vi "gCode_AnalizeAndSend.vi"(9 "UI_Data":T1={"controlTabState"=[], "pathToSTLFiles"=path "", "availableObjs"=[], "objectNames"=[], "addedObjs"=[], "selectedObj"={"Name"="", "objectFiles"=[], "center"={"X"=0.0, "Y"=0.0, "Z"=0.0}, "extent"={"X"=0.0, "Y"=0.0, "Z"=0.0}, "allowedMotion"=enum."XY", "mountOn"=enum."yArm", "Movements"=[], "extraInfo"=[], "hasPOI?"=FALSE, "POI"={"X"=0.0, "Y"=0.0, "Z"=0.0}, "posOffset"={"X"=0.0, "Y"=0.0, "Z"=0.0}, "referenceNum"=refnum}, "3DPictureObjRef"=refnum, "yPOI_0"={"X"=0.0, "Y"=0.0, "Z"=0.0}, "yPOI"={"X"=0.0, "Y"=0.0, "Z"=0.0}, "yPOI_Added?"=FALSE, "breadBoard_00"={"X"=0.0, "Y"=0.0, "Z"=0.0}, "breadBoardOriginOffset"={"X"=0.0, "Y"=0.0, "Z"=0.0}, "XYtranslateObjControls"=[], "ZtranslateObjControls"=[], "pBot_controls"=[], "pBot_VISA"="", "commandLog"="", "pBotConnected?"=FALSE, "pBot_currentEEPROMsettings"="", "realTimeInfoControls"=[], "pBot_tempSensor1"=0.0, "pBot_tempSensor2"=0.0, "realTimeInfoTextColor"=[], "disconnectPBot_Event"=refnum, "needToHomeY?"=FALSE, "pBot_relativePositioning"=FALSE, "pBot_minPos"={"X"=0.0, "Y"=0.0, "Z"=0.0}, "pBot_maxPos"={"X"=0.0, "Y"=0.0, "Z"=0.0}, "pBot_homeOffset"={"X"=0.0, "Y"=0.0, "Z"=0.0}, "textColorGreen"=9174826, "textColorRed"=16750216, "textColorGray"=9868950, "transVisualizationControls"=[], "needToHomeXY?"=FALSE, "pBot_minScanRegion"={"X"=0.0, "Y"=0.0, "Z"=0.0}, "pBot_maxScanRegion"={"X"=0.0, "Y"=0.0, "Z"=0.0}, "pBot_scanN"={"X"=0, "Y"=0, "Z"=0}, "connectedInstruments"=[], "isScanning?"=FALSE, "Wavelengths"=[], "usb2000p_controlRefs"=[], "3DPictureRef"=refnum}, 10 "Input String":string, 11 "Equip_Queue":refnum<queue>) -> (0 "errorOut":errorcluster, 1 "UI_Data out":T1={"controlTabState"=[], "pathToSTLFiles"=path "", "availableObjs"=[], "objectNames"=[], "addedObjs"=[], "selectedObj"={"Name"="", "objectFiles"=[], "center"={"X"=0.0, "Y"=0.0, "Z"=0.0}, "extent"={"X"=0.0, "Y"=0.0, "Z"=0.0}, "allowedMotion"=enum."XY", "mountOn"=enum."yArm", "Movements"=[], "extraInfo"=[], "hasPOI?"=FALSE, "POI"={"X"=0.0, "Y"=0.0, "Z"=0.0}, "posOffset"={"X"=0.0, "Y"=0.0, "Z"=0.0}, "referenceNum"=refnum}, "3DPictureObjRef"=refnum, "yPOI_0"={"X"=0.0, "Y"=0.0, "Z"=0.0}, "yPOI"={"X"=0.0, "Y"=0.0, "Z"=0.0}, "yPOI_Added?"=FALSE, "breadBoard_00"={"X"=0.0, "Y"=0.0, "Z"=0.0}, "breadBoardOriginOffset"={"X"=25.4, "Y"=12.7, "Z"=12.7}, "XYtranslateObjControls"=[], "ZtranslateObjControls"=[], "pBot_controls"=[], "pBot_VISA"="", "commandLog"="", "pBotConnected?"=FALSE, "pBot_currentEEPROMsettings"="", "realTimeInfoControls"=[], "pBot_tempSensor1"=0.0, "pBot_tempSensor2"=0.0, "realTimeInfoTextColor"=[], "disconnectPBot_Event"=refnum, "needToHomeY?"=FALSE, "pBot_relativePositioning"=FALSE, "pBot_minPos"={"X"=0.0, "Y"=0.0, "Z"=0.0}, "pBot_maxPos"={"X"=0.0, "Y"=0.0, "Z"=0.0}, "pBot_homeOffset"={"X"=0.0, "Y"=0.0, "Z"=0.0}, "textColorGreen"=9174826, "textColorRed"=16750216, "textColorGray"=9868950, "transVisualizationControls"=[], "needToHomeXY?"=FALSE, "pBot_minScanRegion"={"X"=0.0, "Y"=0.0, "Z"=0.0}, "pBot_maxScanRegion"={"X"=0.0, "Y"=0.0, "Z"=0.0}, "pBot_scanN"={"X"=0, "Y"=0, "Z"=0}, "connectedInstruments"=[], "isScanning?"=FALSE, "Wavelengths"=[], "usb2000p_controlRefs"=[], "3DPictureRef"=refnum})   [LabVIEW 2015]
uses:
  controls/UI Data.ctl
  processedObjectInfo.ctl
  controls/scanInstrumentInfo.ctl
  support/Message Queue/Message Cluster.ctl
  controls/pBotMessageData.ctl
  support/Message Queue/Enqueue Message (Single).vi
  support/Message Queue/Message Queue.lvlib
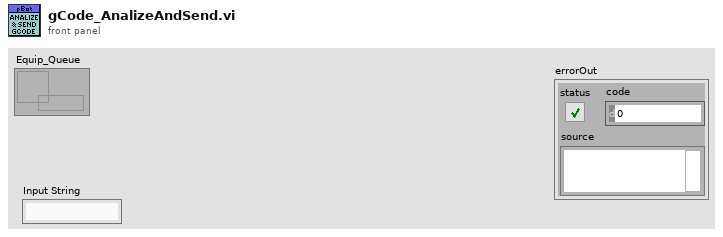
[diagram p1: front panel]
types:
  T1 = typedef "UI Data.ctl" = cluster{"controlTabState":bool[], "pathToSTLFiles":path, "availableObjs":T2[], "objectNames":string[], "addedObjs":T2[], "selectedObj":T2, "3DPictureObjRef":refnum<vi>, "yPOI_0":cluster{"X":dbl, "Y":dbl, "Z":dbl}, "yPOI":cluster{"X":dbl, "Y":dbl, "Z":dbl}, "yPOI_Added?":bool, "breadBoard_00":cluster{"X":dbl, "Y":dbl, "Z":dbl}, "breadBoardOriginOffset":cluster{"X":dbl, "Y":dbl, "Z":dbl}, "XYtranslateObjControls":refnum<vi>[], "ZtranslateObjControls":refnum<vi>[], "pBot_controls":refnum<vi>[], "pBot_VISA":refnum<visa-resource-name>, "commandLog":string, "pBotConnected?":bool, "pBot_currentEEPROMsettings":string, "realTimeInfoControls":refnum<vi>[], "pBot_tempSensor1":dbl, "pBot_tempSensor2":dbl, "realTimeInfoTextColor":u32[], "disconnectPBot_Event":refnum<user-event>, "needToHomeY?":bool, "pBot_relativePositioning":bool, "pBot_minPos":cluster{"X":dbl, "Y":dbl, "Z":dbl}, "pBot_maxPos":cluster{"X":dbl, "Y":dbl, "Z":dbl}, "pBot_homeOffset":cluster{"X":dbl, "Y":dbl, "Z":dbl}, "textColorGreen":u32, "textColorRed":u32, "textColorGray":u32, "transVisualizationControls":refnum<vi>[], "needToHomeXY?":bool, "pBot_minScanRegion":cluster{"X":sgl, "Y":sgl, "Z":sgl}, "pBot_maxScanRegion":cluster{"X":sgl, "Y":sgl, "Z":sgl}, "pBot_scanN":cluster{"X":u16, "Y":u16, "Z":u16}, "connectedInstruments":T3[], "isScanning?":bool, "Wavelengths":dbl[], "usb2000p_controlRefs":refnum<vi>[], "3DPictureRef":refnum<vi>}
  T2 = typedef "processedObjectInfo.ctl" = cluster{"Name":string, "objectFiles":cluster{"Location":path, "Color":cluster{"R":dbl, "G":dbl, "B":dbl, "A":dbl}}[], "center":cluster{"X":dbl, "Y":dbl, "Z":dbl}, "extent":cluster{"X":dbl, "Y":dbl, "Z":dbl}, "allowedMotion":enum16{"XY", "Z"}, "mountOn":enum16{"yArm", "breadBoard"}, "Movements":cluster{"Type":enum16{"rr", "ra", "tr", "ta"}, "vector":cluster{"X":dbl, "Y":dbl, "Z":dbl}, "scalar":dbl}[], "extraInfo":cluster{"parameter":string, "dataType":string, "vector":cluster{"X":dbl, "Y":dbl, "Z":dbl}, "scalar":dbl}[], "hasPOI?":bool, "POI":cluster{"X":dbl, "Y":dbl, "Z":dbl}, "posOffset":cluster{"X":dbl, "Y":dbl, "Z":dbl}, "referenceNum":refnum<vi>}
  T3 = typedef "scanInstrumentInfo.ctl" = cluster{"Name":string, "VISAname":refnum<visa-resource-name>, "1D_dataArraySize":u16, "extraInfo":variant, "error":errorcluster}
  T4 = typedef "pBotMessageData.ctl" = cluster{"commandID":string, "gCode":string, "extraInfo":string, "originatingCommandID":string, "error":errorcluster}
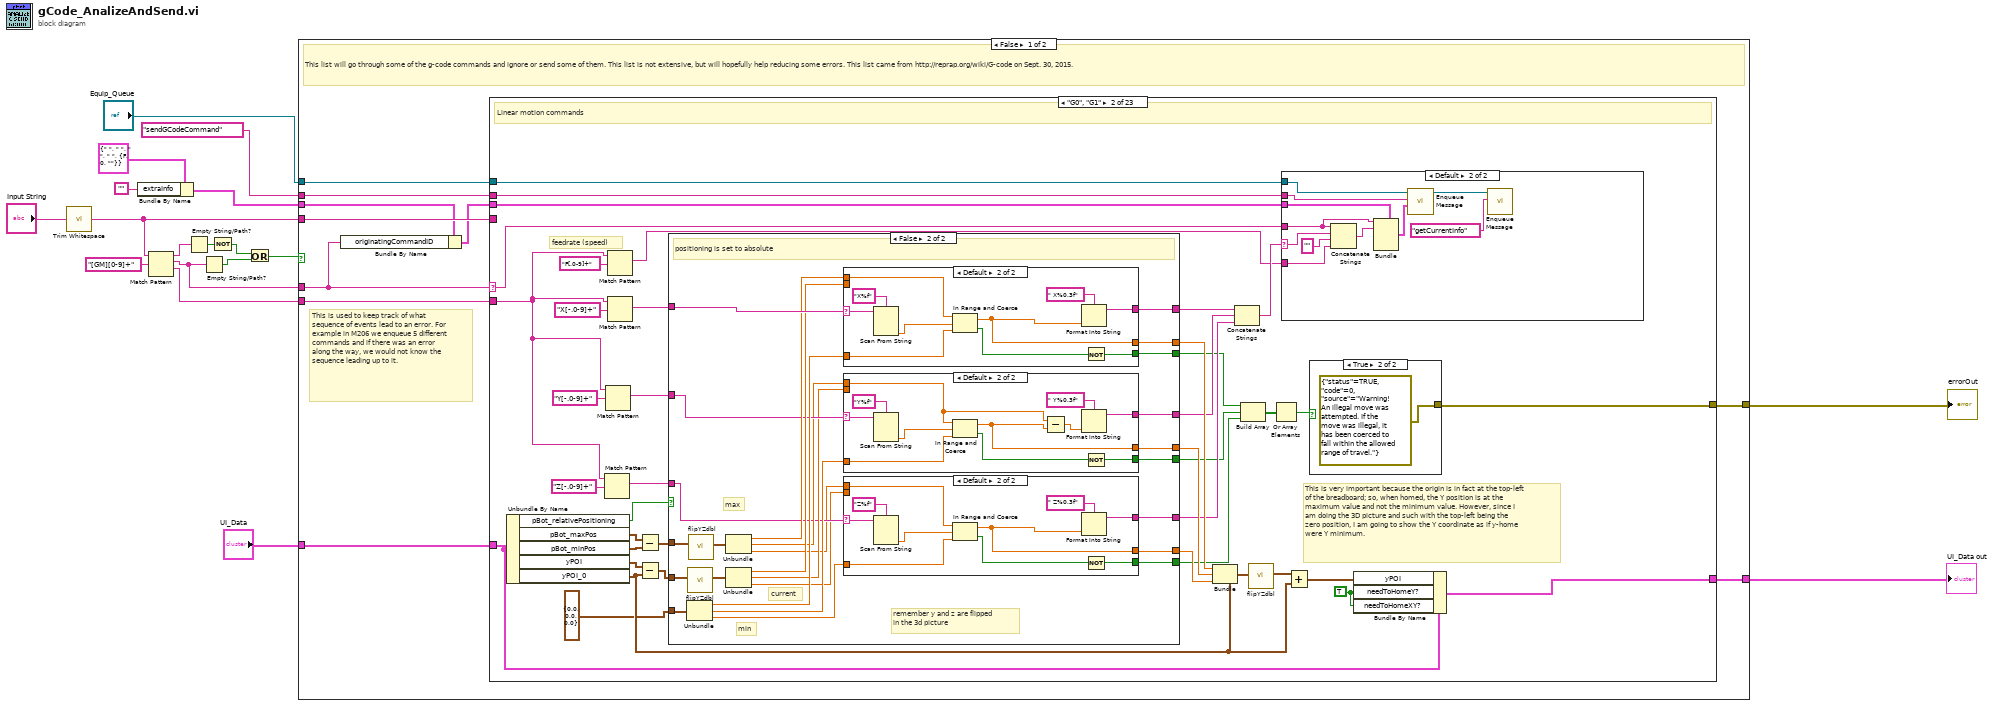
[diagram p0: block diagram]
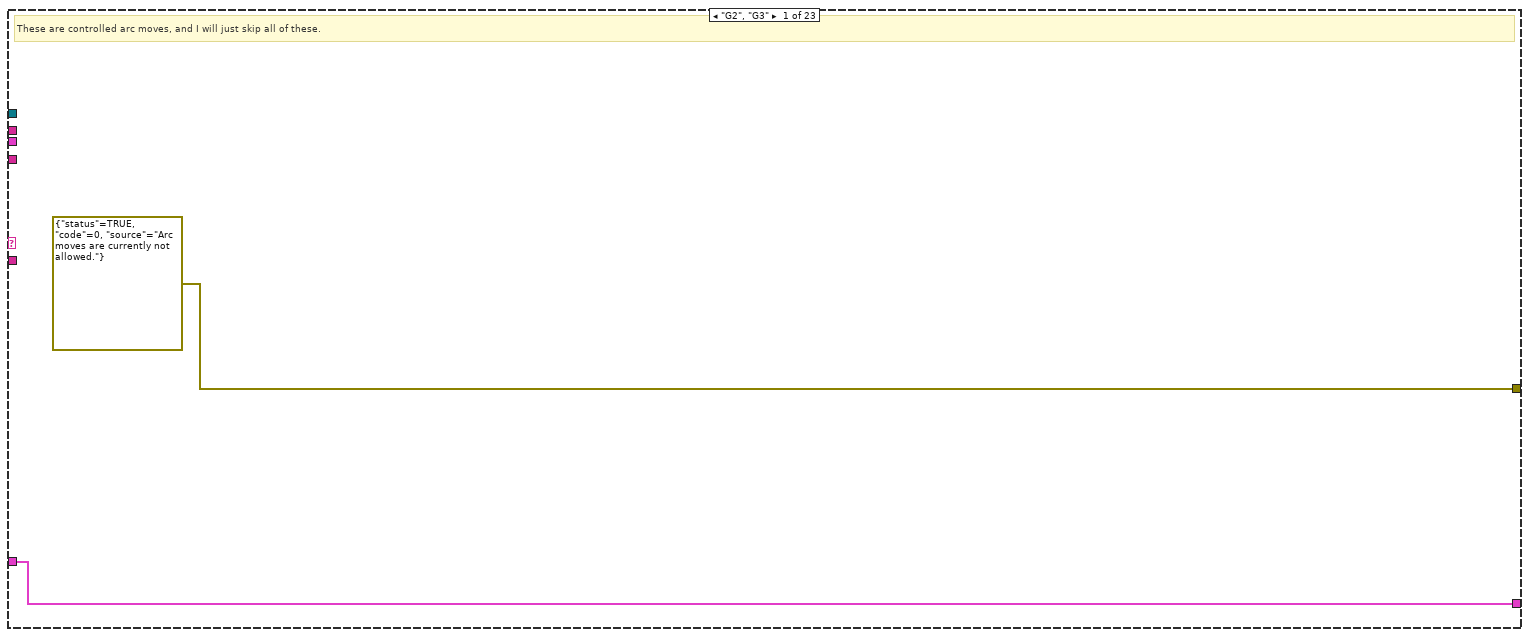
[diagram p2: hidden frame]
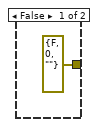
[diagram p3: hidden frame]
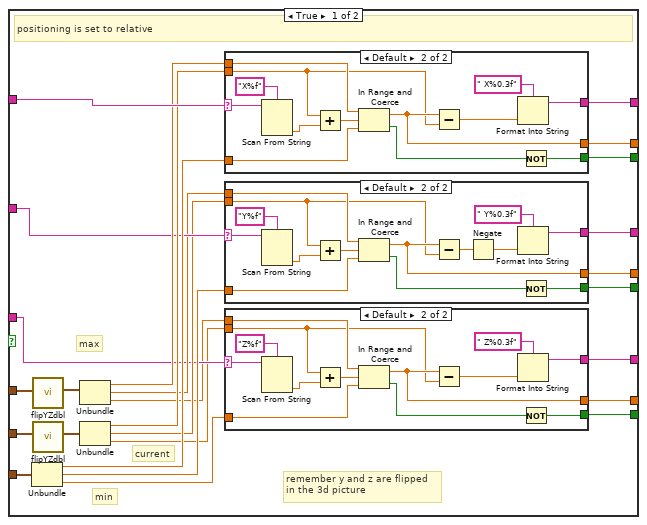
[diagram p5: hidden frame]
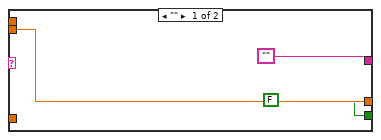
[diagram p6: hidden frame]
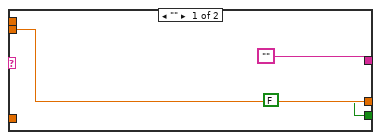
[diagram p7: hidden frame]
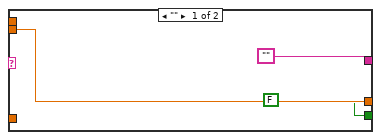
[diagram p8: hidden frame]
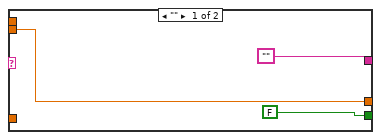
[diagram p9: hidden frame]
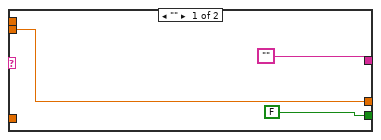
[diagram p10: hidden frame]
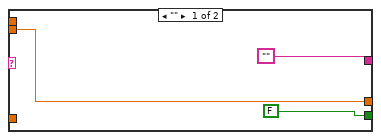
[diagram p11: hidden frame]
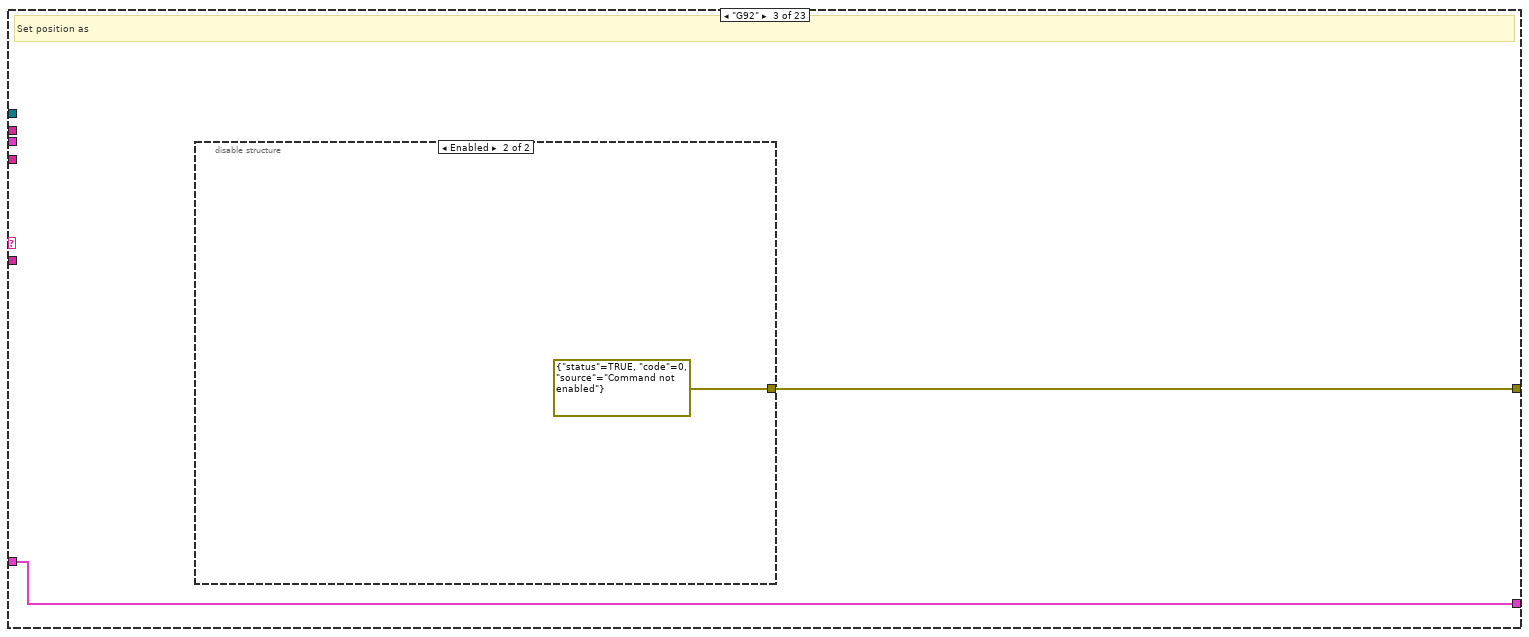
[diagram p12: hidden frame]
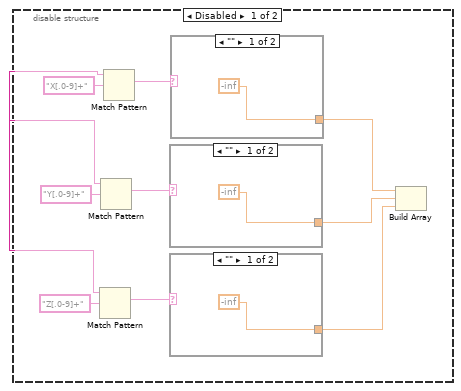
[diagram p13: hidden frame]
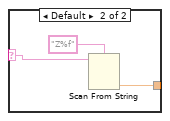
[diagram p14: hidden frame]
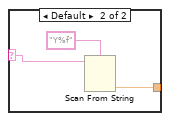
[diagram p15: hidden frame]
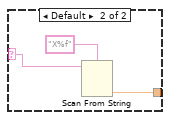
[diagram p16: hidden frame]
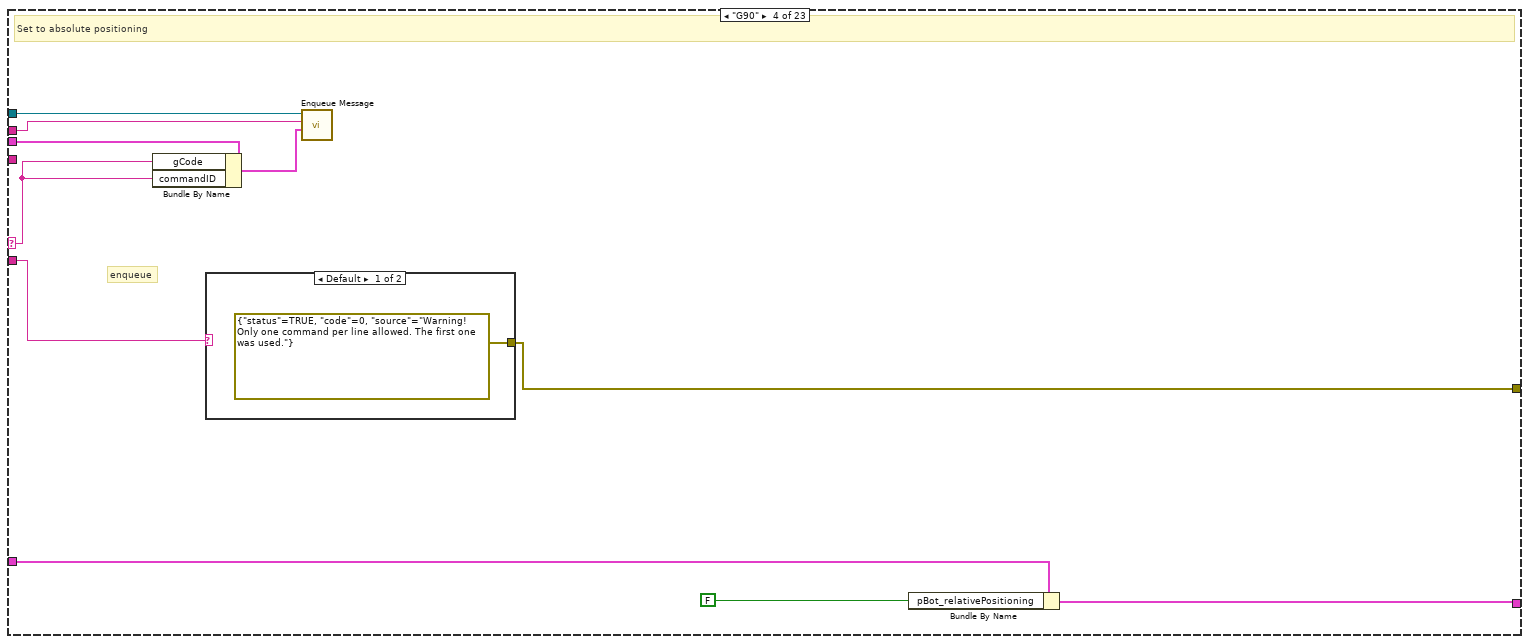
[diagram p17: hidden frame]
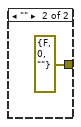
[diagram p18: hidden frame]
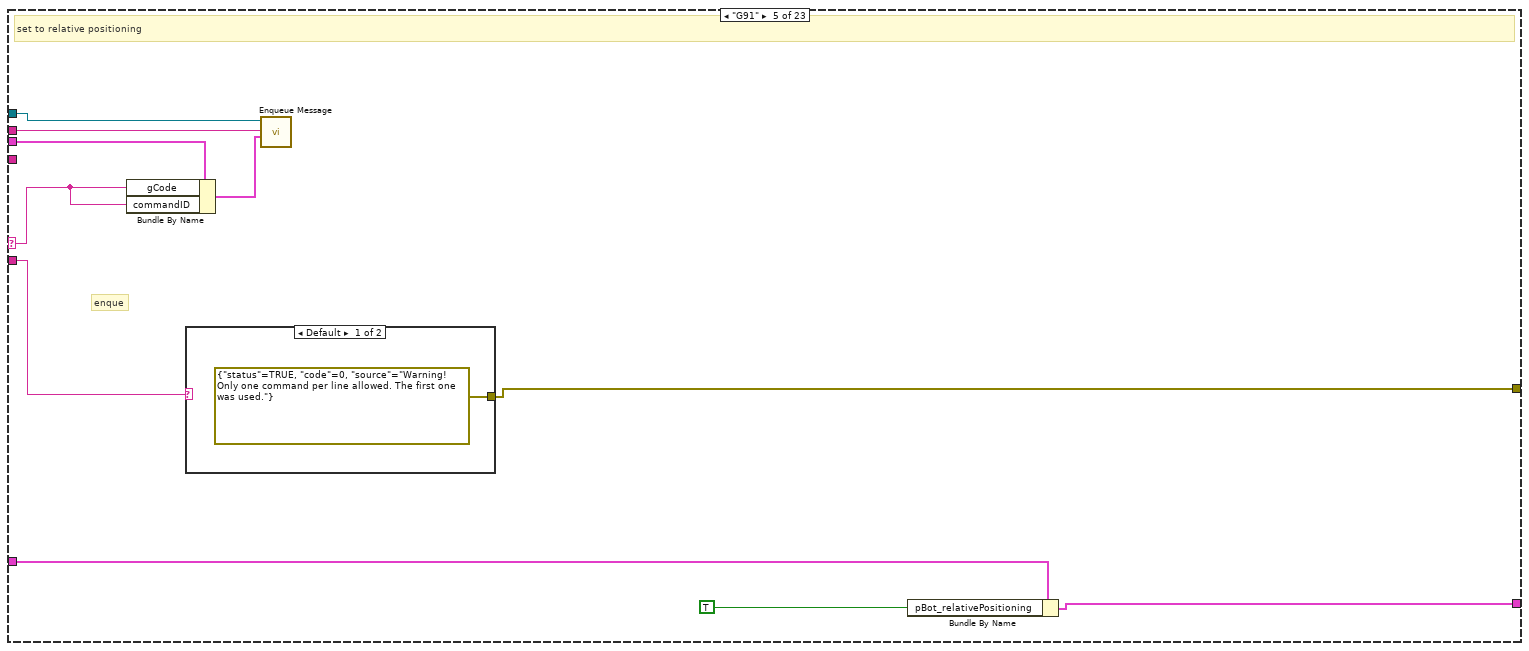
[diagram p19: hidden frame]
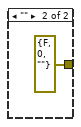
[diagram p20: hidden frame]
diagram:
  n1 = call <vilib>:"Trim Whitespace.vi"("string"="Input String") -> ("trimmed string"=w9:string)  [unwired: 1 in]
  n2 = Bundle By Name(cluster=T4 {"commandID"=" ", "gCode"=" ", "extraInfo"=" ", "originatingCommandID"=" ", "error"={"status"=FALSE, "code"=0, "source"=""}}, "extraInfo"="") -> (w1:T4)
  n3 = Match Pattern(string=w9, regular expression="[GM][0-9]+") -> (before substring=w16:string, match substring=w11:string, after substring=w10:string)  [unwired: 1 in, 1 out]
  n4 = Empty String/Path?(string/path=w16) -> (empty?=w15:bool)
  n5 = Empty String/Path?(string/path=w11) -> (empty?=w13:bool)
  n6 = Not(x=w15) -> (.not. x?=w14:bool)
  n7 = Or(x=w14, y=w13) -> (x .or. y?=w12:bool)
  n8 = case shown="False" w12 {
    tunnel: w11 -> [w19 _]
    tunnel: w10 -> [w28 _]
    tunnel: w9 -> [w27 _]
    tunnel: "UI_Data" -> [w26 w613]
    tunnel: [w25 w613] -> w7
    tunnel: [w24 errorcluster {"status"=TRUE, "code"=0, "source"="Illegal g-code command. The only, currently allowable, commands must begin with either G or M."} ("error constant")] -> w6
    tunnel: "Equip_Queue" -> [w23 _]
    tunnel: "sendGCodeCommand" ("T button name (\"OK\")") -> [w22 _]
    tunnel: w1 -> [w21 _]
    frame False {
      # "This is used to keep track of what sequence of events lead to an error. For example in M206 we enqueue 5 different commands and if there was an error along the way, we would not know the sequence leading up to it."
      # "This list will go through some of the g-code commands and ignore or send some of them. This list is not extensive, but will hopefully help reducing some errors. This list came from http://reprap.org/wiki/G-code on Sept. 30, 2015."
      n9 = Bundle By Name(cluster=w21, "originatingCommandID"=w19) -> (w20:T4)
      n10 = case shown="\"G0\", \"G1\"" w19 {
        selector: w19 -> [_ w55 _ w250 w262 _ _ _ _ w354 _ _ w368 _ w408 _ w484 w547 w559 w575 w585 _ w597]
        tunnel: [errorcluster {"status"=TRUE, "code"=0, "source"="Arc moves are currently not allowed."} ("error constant") w48 w226 w255 w269 errorcluster {"status"=TRUE, "code"=0, "source"="Auto-leveling not supported"} ("error constant") w276 errorcluster {"status"=TRUE, "code"=0, "source"="SD card functionality not supported"} ("error constant") errorcluster {"status"=TRUE, "code"=0, "source"="There is no extruder."} ("error constant") w360 errorcluster {"status"=TRUE, "code"=0, "source"="No fan installed."} ("error constant") errorcluster {"status"=TRUE, "code"=0, "source"="Ignored"} ("error constant") w374 errorcluster {"status"=TRUE, "code"=0, "source"="No heated bed installed."} ("error constant") w380 errorcluster {"status"=TRUE, "code"=0, "source"="This is a dependent property and cannot be set. This property is given by the negative of the home offset (M206)."} ("error constant") _ _ w557 w581 w591 errorcluster {"status"=TRUE, "code"=0, "source"="ignored"} ("error constant") _] -> w24
        tunnel: w28 -> [_ w46 _ w256 w270 _ w281 _ _ w361 _ _ w375 _ w412 _ w485 _ w558 w582 w592 _ _]
        tunnel: w27 -> [_ _ _ _ _ _ _ _ _ _ _ _ _ _ w411 _ _ w548 _ _ _ _ w602]
        tunnel: w26 -> [w29 w63 w225 w259 w268 w274 w280 w350 w352 w359 w364 w366 w373 w378 w407 w474 w480 w552 w556 w580 w590 w595 w601]
        tunnel: [w29 w54 w225 w257 w267 w274 w280 w350 w352 w359 w364 w366 w373 w378 w407 w474 w480 w552 w556 w580 w590 w595 w601] -> w25
        tunnel: w23 -> [_ w44 _ w254 w263 _ w279 _ _ w355 _ _ w372 _ w409 _ w481 w551 w553 w578 w586 _ w600]
        tunnel: w22 -> [_ w43 _ w253 w264 _ w278 _ _ w356 _ _ w371 _ w410 _ w482 w550 w554 w577 w587 _ w599]
        tunnel: w20 -> [_ w42 _ w252 w266 _ w277 _ _ w357 _ _ w370 _ w406 _ w483 w549 w555 w576 w589 _ w598]
        frame "G2", "G3" {
          # "These are controlled arc moves, and I will just skip all of these."
        }
        frame "G0", "G1" {
          w31 = TRUE ("needToHomeY?")
          # "This is very important because the origin is in fact at the top-left of the breadboard; so, when homed, the Y position is at the maximum value and not the minimum value. However, since I am doing the 3D picture and such with the top-left being the zero position, I am going to show the Y coordinate as if y-home were Y minimum."
          # "feedrate (speed)"
          # "Linear motion commands"
          n11 = Unbundle By Name(w63) -> ("pBot_relativePositioning"=w64:bool, "pBot_maxPos"=w35:cluster{"X":dbl, "Y":dbl, "Z":dbl}, "pBot_minPos"=w34:cluster{"X":dbl, "Y":dbl, "Z":dbl}, "yPOI"=w41:cluster{"X":dbl, "Y":dbl, "Z":dbl}, "yPOI_0"=w39:cluster{"X":dbl, "Y":dbl, "Z":dbl})
          n12 = Match Pattern(string=w46, regular expression="Z[-.0-9]+") -> (match substring=w70:string)  [unwired: 1 in, 3 out]
          n13 = Match Pattern(string=w46, regular expression="Y[-.0-9]+") -> (match substring=w69:string)  [unwired: 1 in, 3 out]
          n14 = Match Pattern(string=w46, regular expression="F[.0-9]+") -> (match substring=w45:string)  [unwired: 1 in, 3 out]
          n15 = Match Pattern(string=w46, regular expression="X[-.0-9]+") -> (match substring=w68:string)  [unwired: 1 in, 3 out]
          n16 = Subtract(x=w35, y=w34) -> (x-y=w33:cluster{"X":dbl, "Y":dbl, "Z":dbl})
          n17 = Subtract(x=w41, y=w39) -> (x-y=w40:cluster{"X":dbl, "Y":dbl, "Z":dbl})
          n18 = case shown="False" w64 {
            tunnel: w70 -> [w92 w167]
            tunnel: w69 -> [w99 w174]
            tunnel: w68 -> [w109 w184]
            tunnel: w33 -> [w84 w160]
            tunnel: w40 -> [w104 w179]
            tunnel: cluster{"X":dbl, "Y":dbl, "Z":dbl} {"X"=0.0, "Y"=0.0, "Z"=0.0} ("pBot_minPos") -> [w108 w183]
            tunnel: [w102 w177] -> w59
            tunnel: [w101 w176] -> w62
            tunnel: [w95 w170] -> w58
            tunnel: [w94 w169] -> w61
            tunnel: [w88 w163] -> w57
            tunnel: [w87 w162] -> w60
            tunnel: [w100 w175] -> w52
            tunnel: [w93 w168] -> w51
            tunnel: [w86 w161] -> w50
            frame True {
              # "remember y and z are flipped\nin the 3d picture"
              # "min"
              # "current"
              # "max"
              # "positioning is set to relative"
              n19 = Unbundle(w108) -> ("X"=w105:dbl, "Y"=w96:dbl, "Z"=w89:dbl)
              n20 = call "flipYZdbl.vi"("pointIn"=w84) -> ("pointOut"=w85:cluster{"X":dbl, "Y":dbl, "Z":dbl})  [unwired: 10 in]
              n21 = call "flipYZdbl.vi"("pointIn"=w104) -> ("pointOut"=w103:cluster{"X":dbl, "Y":dbl, "Z":dbl})  [unwired: 10 in]
              n22 = Unbundle(w85) -> ("X"=w107:dbl, "Y"=w98:dbl, "Z"=w91:dbl)
              n23 = Unbundle(w103) -> ("X"=w106:dbl, "Y"=w97:dbl, "Z"=w90:dbl)
              n24 = case shown="Default" w109 {
                selector: w109 -> [_ w157]
                tunnel: w107 -> [_ w154]
                tunnel: w106 -> [w144 w146]
                tunnel: w105 -> [_ w155]
                tunnel: ["" w153] -> w102
                tunnel: [w144 w152] -> w101
                tunnel: [FALSE w151] -> w100
                frame "" {
                }
                frame Default {
                  n25 = Scan From String(format string="X%f", input string=w157) -> (output 1=w147:dbl)  [unwired: 3 in, 3 out]
                  n26 = Add(x=w146, y=w147) -> (x+y=w156:dbl)
                  n27 = In Range and Coerce(upper limit=w154, x=w156, lower limit=w155) -> (coerced(x)=w152:dbl, In Range?=w150:bool)
                  n28 = Subtract(x=w152, y=w146) -> (x-y=w149:dbl)
                  n29 = Format Into String(format string=" X%0.3f", w149) -> (resulting string=w153:string)  [unwired: 2 in, 1 out]
                  n30 = Not(x=w150) -> (.not. x?=w151:bool)
                }
              }
              n31 = case shown="Default" w99 {
                selector: w99 -> [_ w141]
                tunnel: w98 -> [_ w138]
                tunnel: w97 -> [w127 w131]
                tunnel: w96 -> [_ w139]
                tunnel: ["" w137] -> w95
                tunnel: [w127 w136] -> w94
                tunnel: [FALSE w135] -> w93
                frame "" {
                }
                frame Default {
                  n32 = Scan From String(format string="Y%f", input string=w141) -> (output 1=w132:dbl)  [unwired: 3 in, 3 out]
                  n33 = Add(x=w131, y=w132) -> (x+y=w140:dbl)
                  n34 = In Range and Coerce(upper limit=w138, x=w140, lower limit=w139) -> (coerced(x)=w136:dbl, In Range?=w134:bool)
                  n35 = Subtract(x=w136, y=w131) -> (x-y=w130:dbl)
                  n36 = Negate(x=w130) -> (-x=w129:dbl)
                  n37 = Format Into String(format string=" Y%0.3f", w129) -> (resulting string=w137:string)  [unwired: 2 in, 1 out]
                  n38 = Not(x=w134) -> (.not. x?=w135:bool)
                }
              }
              n39 = case shown="Default" w92 {
                selector: w92 -> [_ w124]
                tunnel: w91 -> [_ w121]
                tunnel: w90 -> [w111 w114]
                tunnel: w89 -> [_ w122]
                tunnel: ["" w120] -> w88
                tunnel: [w111 w119] -> w87
                tunnel: [FALSE w118] -> w86
                frame "" {
                }
                frame Default {
                  n40 = Scan From String(format string="Z%f", input string=w124) -> (output 1=w115:dbl)  [unwired: 3 in, 3 out]
                  n41 = Add(x=w114, y=w115) -> (x+y=w123:dbl)
                  n42 = In Range and Coerce(upper limit=w121, x=w123, lower limit=w122) -> (coerced(x)=w119:dbl, In Range?=w117:bool)
                  n43 = Subtract(x=w119, y=w114) -> (x-y=w113:dbl)
                  n44 = Format Into String(format string=" Z%0.3f", w113) -> (resulting string=w120:string)  [unwired: 2 in, 1 out]
                  n45 = Not(x=w117) -> (.not. x?=w118:bool)
                }
              }
            }
            frame False {
              # "remember y and z are flipped\nin the 3d picture"
              # "min"
              # "current"
              # "max"
              # "positioning is set to absolute"
              n46 = Unbundle(w183) -> ("X"=w180:dbl, "Y"=w171:dbl, "Z"=w164:dbl)
              n47 = call "flipYZdbl.vi"("pointIn"=w179) -> ("pointOut"=w178:cluster{"X":dbl, "Y":dbl, "Z":dbl})  [unwired: 10 in]
              n48 = call "flipYZdbl.vi"("pointIn"=w160) -> ("pointOut"=w159:cluster{"X":dbl, "Y":dbl, "Z":dbl})  [unwired: 10 in]
              n49 = Unbundle(w159) -> ("X"=w182:dbl, "Y"=w173:dbl, "Z"=w166:dbl)
              n50 = Unbundle(w178) -> ("X"=w181:dbl, "Y"=w172:dbl, "Z"=w165:dbl)
              n51 = case shown="Default" w184 {
                selector: w184 -> [_ w223]
                tunnel: w182 -> [_ w221]
                tunnel: w181 -> [w213 _]
                tunnel: w180 -> [_ w222]
                tunnel: ["" w220] -> w177
                tunnel: [w213 w215] -> w176
                tunnel: [FALSE w219] -> w175
                frame "" {
                }
                frame Default {
                  n52 = Scan From String(format string="X%f", input string=w223) -> (output 1=w216:dbl)  [unwired: 3 in, 3 out]
                  n53 = In Range and Coerce(upper limit=w221, x=w216, lower limit=w222) -> (coerced(x)=w215:dbl, In Range?=w218:bool)
                  n54 = Format Into String(format string=" X%0.3f", w215) -> (resulting string=w220:string)  [unwired: 2 in, 1 out]
                  n55 = Not(x=w218) -> (.not. x?=w219:bool)
                }
              }
              n56 = case shown="Default" w174 {
                selector: w174 -> [_ w210]
                tunnel: w173 -> [_ w201]
                tunnel: w172 -> [w199 _]
                tunnel: w171 -> [_ w209]
                tunnel: ["" w208] -> w170
                tunnel: [w199 w202] -> w169
                tunnel: [FALSE w207] -> w168
                frame "" {
                }
                frame Default {
                  n57 = Scan From String(format string="Y%f", input string=w210) -> (output 1=w204:dbl)  [unwired: 3 in, 3 out]
                  n58 = In Range and Coerce(upper limit=w201, x=w204, lower limit=w209) -> (coerced(x)=w202:dbl, In Range?=w206:bool)
                  n59 = Subtract(x=w201, y=w202) -> (x-y=w203:dbl)
                  n60 = Format Into String(format string=" Y%0.3f", w203) -> (resulting string=w208:string)  [unwired: 2 in, 1 out]
                  n61 = Not(x=w206) -> (.not. x?=w207:bool)
                }
              }
              n62 = case shown="Default" w167 {
                selector: w167 -> [_ w196]
                tunnel: w166 -> [_ w194]
                tunnel: w165 -> [w186 _]
                tunnel: w164 -> [_ w195]
                tunnel: ["" w193] -> w163
                tunnel: [w186 w188] -> w162
                tunnel: [FALSE w192] -> w161
                frame "" {
                }
                frame Default {
                  n63 = Scan From String(format string="Z%f", input string=w196) -> (output 1=w189:dbl)  [unwired: 3 in, 3 out]
                  n64 = In Range and Coerce(upper limit=w194, x=w189, lower limit=w195) -> (coerced(x)=w188:dbl, In Range?=w191:bool)
                  n65 = Format Into String(format string=" Z%0.3f", w188) -> (resulting string=w193:string)  [unwired: 2 in, 1 out]
                  n66 = Not(x=w191) -> (.not. x?=w192:bool)
                }
              }
            }
          }
          n67 = Bundle(cluster=w39, "X"=w62, "Y"=w61, "Z"=w60) -> (w37:cluster{"X":dbl, "Y":dbl, "Z":dbl})
          n68 = Concatenate Strings(w59, w58, w57) -> (w56:string)
          n69 = Build Array(w52, w51, w50) -> (w53:bool[])
          n70 = call "flipYZdbl.vi"("pointIn"=w37) -> ("pointOut"=w36:cluster{"X":dbl, "Y":dbl, "Z":dbl})  [unwired: 10 in]
          n71 = Or Array Elements(Boolean array=w53) -> (logical OR=w49:bool)
          n72 = case shown="Default" w56 {
            selector: w56 -> [_ w83]
            tunnel: w55 -> [_ w76]
            tunnel: w45 -> [_ w81]
            tunnel: w44 -> [_ w77]
            tunnel: w43 -> [_ w78]
            tunnel: w42 -> [_ w80]
            frame "" {
            }
            frame Default {
              n73 = Concatenate Strings(w76, w83, "" ("string"), w81) -> (w75:string)
              n74 = Bundle(cluster=w80, "commandID"=w76, "gCode"=w75) -> (w79:T4)  [unwired: 3 in]
              n75 = call-poly "Enqueue Message.vi"("Message Data"=w79, "Message"=w78, "Message Queue"=w77) -> ("dup Message Queue"=w74:refnum<queue>)  [unwired: 7 in, 1 out]
              n76 = call-poly "Enqueue Message.vi"("Message"="getCurrentInfo", "Message Queue"=w74) -> ()  [unwired: 8 in, 2 out]
            }
          }
          n77 = Add(x=w36, y=w39) -> (x+y=w38:cluster{"X":dbl, "Y":dbl, "Z":dbl})
          n78 = case shown="True" w49 {
            tunnel: [errorcluster {"status"=FALSE, "code"=0, "source"=""} ("error constant") errorcluster {"status"=TRUE, "code"=0, "source"="Warning! An illegal move was attempted. If the move was illegal, it has been coerced to fall within the allowed range of travel."} ("error constant")] -> w48
            frame False {
            }
            frame True {
            }
          }
          n79 = Bundle By Name(cluster=w63, "yPOI"=w38, "needToHomeY?"=w31, "needToHomeXY?"=w31) -> (w54:T1)
        }
        frame "G92" {
          # "Set position as"
          n80 = disable-structure shown="Enabled" {
            disable-tunnel: [_ errorcluster {"status"=TRUE, "code"=0, "source"="Command not enabled"} ("error constant")] -> w226
            frame Disabled {
              n81 = Match Pattern(regular expression="X[.0-9]+") -> (string=w230:string, match substring=w234:string)  [unwired: 1 in, 3 out]
              n82 = Match Pattern(string=w230, regular expression="Z[.0-9]+") -> (match substring=w236:string)  [unwired: 1 in, 3 out]
              n83 = Match Pattern(string=w230, regular expression="Y[.0-9]+") -> (match substring=w235:string)  [unwired: 1 in, 3 out]
              n84 = case shown="\"\"" w235 {
                selector: w235 -> [_ w242]
                tunnel: [-inf w243] -> w228
                frame "" {
                }
                frame Default {
                  n85 = Scan From String(format string="Y%f", input string=w242) -> (output 1=w243:dbl)  [unwired: 3 in, 3 out]
                }
              }
              n86 = case shown="\"\"" w236 {
                selector: w236 -> [_ w239]
                tunnel: [-inf w238] -> w227
                frame "" {
                }
                frame Default {
                  n87 = Scan From String(format string="Z%f", input string=w239) -> (output 1=w238:dbl)  [unwired: 3 in, 3 out]
                }
              }
              n88 = case shown="\"\"" w234 {
                selector: w234 -> [_ w247]
                tunnel: [-inf w246] -> w229
                frame "" {
                }
                frame Default {
                  n89 = Scan From String(format string="X%f", input string=w247) -> (output 1=w246:dbl)  [unwired: 3 in, 3 out]
                }
              }
              n90 = Build Array(w229, w228, w227) -> ()  [unwired: 1 out]
            }
            frame Enabled {
            }
          }
        }
        frame "G90" {
          # "enqueue"
          # "Set to absolute positioning"
          n91 = Bundle By Name(cluster=w252, "gCode"=w250, "commandID"=w250) -> (w251:T4)
          n92 = case shown="Default" w256 {
            tunnel: [errorcluster {"status"=TRUE, "code"=0, "source"="Warning! Only one command per line allowed. The first one was used."} ("error constant") errorcluster {"status"=FALSE, "code"=0, "source"=""} ("error constant")] -> w255
            frame Default {
            }
            frame "" {
            }
          }
          n93 = call-poly "Enqueue Message.vi"("Message Data"=w251, "Message"=w253, "Message Queue"=w254) -> ()  [unwired: 7 in, 2 out]
          n94 = Bundle By Name(cluster=w259, "pBot_relativePositioning"=FALSE) -> (w257:T1)
        }
        frame "G91" {
          # "enque"
          # "set to relative positioning"
          n95 = Bundle By Name(cluster=w266, "gCode"=w262, "commandID"=w262) -> (w265:T4)
          n96 = case shown="Default" w270 {
            tunnel: [errorcluster {"status"=TRUE, "code"=0, "source"="Warning! Only one command per line allowed. The first one was used."} ("error constant") errorcluster {"status"=FALSE, "code"=0, "source"=""} ("error constant")] -> w269
            frame Default {
            }
            frame "" {
            }
          }
          n97 = call-poly "Enqueue Message.vi"("Message Data"=w265, "Message"=w264, "Message Queue"=w263) -> ()  [unwired: 7 in, 2 out]
          n98 = Bundle By Name(cluster=w268, "pBot_relativePositioning"=TRUE) -> (w267:T1)
        }
        frame "G29" {
          # "This command would measure the position of the bed in three positions and then fit those points to a plane. Using this plane, the firmware would correct for any unlevelness of the bed in real time. However, since the bed is not metal and the curent position of the probe is off the bed; this command is not allowed.\nAt some time, we should make a head mount to hold the z-sensor, and then put aluminum foil on the bed so that we can use this command. However, you would not want to do this everytime you turn the printer on, and I do not know if the values it measured are stored in the onboard memory between reboots and if it would automatically use the values. (In 3D printing this command is run betore every single 3d print and so it doesnt need to be stored.)"
        }
        frame "G28" {
          # "Home the axis -- note we need to home Y first then X and then Z. This is to reduce the posibitlity of the head colliding with any objects on the breadboard."
          n99 = disable-structure shown="Enabled" {
            disable-tunnel: w281 -> [w286 _]
            disable-tunnel: w279 -> [w285 _]
            disable-tunnel: w278 -> [w284 _]
            disable-tunnel: w277 -> [w283 _]
            disable-tunnel: [errorcluster {"status"=FALSE, "code"=0, "source"=""} ("error constant") errorcluster {"status"=TRUE, "code"=0, "source"="Diabled use the home buttons"} ("error constant")] -> w276
            frame Disabled {
              n100 = case shown="\"\"" w286 {
                selector: w286 -> [w290 _]
                tunnel: w285 -> [w287 w331]
                tunnel: w284 -> [w288 w332]
                tunnel: w283 -> [w289 w333]
                frame Default {
                  # "search for the axis to home and then enque new sendGCodeCommand messages to home the axis individualy and in the proper time"
                  n101 = stacked-sequence {
                    tunnel: w290 -> [w295 w307 w319 _]
                    tunnel: w289 -> [w293 w305 w317 _]
                    tunnel: w288 -> [w292 w304 w316 _]
                    tunnel: w287 -> [w291 w303 w315 w327]
                    frame #0 {
                      n102 = Match Pattern(string=w295, regular expression="Y") -> (match substring=w294:string)  [unwired: 1 in, 3 out]
                      n103 = case shown="Default" w294 {
                        tunnel: w293 -> [_ w300]
                        tunnel: w292 -> [_ w299]
                        tunnel: w291 -> [_ w298]
                        frame "" {
                        }
                        frame Default {
                          # "enqueue"
                          n104 = Bundle By Name(cluster=w300, "gCode"="G28 Y" ("regular expression"), "commandID"="homeY" ("regular expression")) -> (w297:T4)
                          n105 = call-poly "Enqueue Message.vi"("Message Data"=w297, "Message"=w299, "Message Queue"=w298) -> ()  [unwired: 7 in, 2 out]
                        }
                      }
                    }
                    frame #1 {
                      n106 = Match Pattern(string=w307, regular expression="X") -> (match substring=w306:string)  [unwired: 1 in, 3 out]
                      n107 = case shown="Default" w306 {
                        tunnel: w305 -> [_ w312]
                        tunnel: w304 -> [_ w311]
                        tunnel: w303 -> [_ w310]
                        frame "" {
                        }
                        frame Default {
                          # "enqueue"
                          n108 = Bundle By Name(cluster=w312, "gCode"="G28 X" ("regular expression"), "commandID"="homeX" ("regular expression")) -> (w309:T4)
                          n109 = call-poly "Enqueue Message.vi"("Message Data"=w309, "Message"=w311, "Message Queue"=w310) -> ()  [unwired: 7 in, 2 out]
                        }
                      }
                    }
                    frame #2 {
                      n110 = Match Pattern(string=w319, regular expression="Z") -> (match substring=w318:string)  [unwired: 1 in, 3 out]
                      n111 = case shown="Default" w318 {
                        tunnel: w317 -> [_ w324]
                        tunnel: w316 -> [_ w323]
                        tunnel: w315 -> [_ w322]
                        frame "" {
                        }
                        frame Default {
                          # "enqueue"
                          n112 = Bundle By Name(cluster=w324, "gCode"="G28 Z" ("regular expression"), "commandID"="homeZ" ("regular expression")) -> (w321:T4)
                          n113 = call-poly "Enqueue Message.vi"("Message Data"=w321, "Message"=w323, "Message Queue"=w322) -> ()  [unwired: 7 in, 2 out]
                        }
                      }
                    }
                    frame #3 {
                      n114 = call-poly "Enqueue Message.vi"("Message"="getCurrentInfo", "Message Queue"=w327) -> ()  [unwired: 8 in, 2 out]
                    }
                  }
                }
                frame "" {
                  # "enqueue these items"
                  # "Home all axis -- G28 by itself seems to do something wierd when it tryed to home the Z axis, plus it homes the X axis first. Thus, I will just send three messages: home y, home x, home z"
                  n115 = Build Array("homeY", "homeX", "homeZ") -> (w334:string[])
                  n116 = Build Array("G28 Y", "G28 X", "G28 Z") -> (w338:string[])
                  n117 = for {
                    tunnel: w338 -> [w348] mode=indexing
                    tunnel: w334 -> [w347] mode=indexing
                    tunnel: w333 -> [w345]
                    tunnel: w332 -> [w344]
                    tunnel: w331 -> [w343]
                    tunnel: [w342] -> w329
                    n118 = Bundle By Name(cluster=w345, "gCode"=w348, "commandID"=w347) -> (w346:T4)
                    n119 = call-poly "Enqueue Message.vi"("Message Data"=w346, "Message"=w344, "Message Queue"=w343) -> ("dup Message Queue"=w342:refnum<queue>)  [unwired: 7 in, 1 out]
                  }
                  n120 = call-poly "Enqueue Message.vi"("Message"="getCurrentInfo", "Message Queue"=w329) -> ()  [unwired: 8 in, 2 out]
                }
              }
            }
            frame Enabled {
            }
          }
        }
        frame "M20", "M21", "M22", "M23", "M24", "M25", "M26", "M27", "M28", "M29", "M30", "M31", "M32", "M33", "M34", "M928" {
          # "These commands are all about SD cards and will be ignored."
        }
        frame "M104", "M108", "M109", "M207", "M221", "M82", "M83" {
          # "Commands about extruders that will be ignored.\nNote --- M83, M109 are about setting the temperature of the extruder. If a heater was installed (for instance for cell incumation) and the correct thermistor was used for measuring the temperature, then this command might be able to be used for setting that temperature."
        }
        frame "M105" {
          # "enqueue"
          # "Get current extruder/bed temperature"
          n121 = Bundle By Name(cluster=w357, "commandID"=w354, "gCode"=w354) -> (w358:T4)
          n122 = case shown="Default" w361 {
            tunnel: [errorcluster {"status"=TRUE, "code"=0, "source"="Warning! Only one command per line allowed. The first one was used."} ("error constant") errorcluster {"status"=FALSE, "code"=0, "source"=""} ("error constant")] -> w360
            frame Default {
            }
            frame "" {
            }
          }
          n123 = call-poly "Enqueue Message.vi"("Message Data"=w358, "Message"=w356, "Message Queue"=w355) -> ()  [unwired: 7 in, 2 out]
        }
        frame "M106", "M107" {
          # "Turn fan on or off. -- currently no fan installed"
        }
        frame "M112" {
          # "I don't know if I should do this or not, and I dont want to test it; so, for now it will be disabled"
          # "Emergancy stop. All moves immediately terminated, then all motors and heaters are turned off. To start again, need to press the master reset button on the printerBoard (says wikipedia -- never tried this command though."
        }
        frame "M114" {
          # "enque"
          # "Get current position."
          n124 = Bundle By Name(cluster=w370, "commandID"=w368, "gCode"=w368) -> (w369:T4)
          n125 = case shown="\"\"" w375 {
            tunnel: [errorcluster {"status"=TRUE, "code"=0, "source"="Warning! Only one command per line allowed. The first one was used."} ("error constant") errorcluster {"status"=FALSE, "code"=0, "source"=""} ("error constant")] -> w374
            frame Default {
            }
            frame "" {
            }
          }
          n126 = call-poly "Enqueue Message.vi"("Message Data"=w369, "Message"=w371, "Message Queue"=w372) -> ()  [unwired: 7 in, 2 out]
        }
        frame "M140", "M190" {
          # "Commands for setting temperature of heated bed -- no heated bed installed"
        }
        frame "M206" {
          # "travel range"
          # "Note! I will actually disable the user from being able to modify this value.\nInstead I need to make a new option called set home_Offset and then maybe prompt the user for the values between the current yPOI and the 0,0 hole of the breadBoard. Then using the known offsets of the yPOI I will calculate what the home offset should be."
          # "Set home offset. Essentially I do not want a home offset. When we home all of the axis, I want the position to be 0,0,0 (well its actually 0,max(y),0). However, I also want to save the offset position of the yArm to the breadboard in the hardware so that I do not need a seperate file to save settings in. Thus, I will use the home offset to store this offset between the yArm and the breadboard and I will subtract this same offset from the minimum and maximum position so that everything still works well. (The way the printer works is that the home position is the minimum position plus the home offset; so the (min pos) = -(home offset). Also, I still want [(max pos) - (min pos)] = travel range, so (max pos) = (travel range) + (min pos) = (travel range) - (home offset)"
          n127 = Unbundle By Name(w407) -> ("pBot_maxPos"=w401:cluster{"X":dbl, "Y":dbl, "Z":dbl}, "pBot_minPos"=w400:cluster{"X":dbl, "Y":dbl, "Z":dbl})
          n128 = Subtract(x=w401, y=w400) -> (x-y=w398:cluster{"X":dbl, "Y":dbl, "Z":dbl})
          n129 = Match Pattern(string=w412, regular expression="Z[-.0-9]+") -> (match substring=w394:string)  [unwired: 1 in, 3 out]
          n130 = Match Pattern(string=w412, regular expression="Y[-.0-9]+") -> (match substring=w393:string)  [unwired: 1 in, 3 out]
          n131 = Match Pattern(string=w412, regular expression="X[-.0-9]+") -> (match substring=w399:string)  [unwired: 1 in, 3 out]
          n132 = call "flipYZdbl.vi"("pointIn"=w398) -> ("pointOut"=w397:cluster{"X":dbl, "Y":dbl, "Z":dbl})  [unwired: 10 in]
          n133 = Unbundle(w397) -> ("X"=w402:dbl, "Y"=w396:dbl, "Z"=w395:dbl)
          n134 = case shown="Default" w393 {
            selector: w393 -> [_ w460]
            tunnel: w396 -> [_ w458]
            tunnel: [w451 w459] -> w387
            tunnel: [w451 w453] -> w384
            tunnel: [errorcluster {"status"=TRUE, "code"=0, "source"=""} ("error constant") errorcluster {"status"=FALSE, "code"=0, "source"=""} ("error constant")] -> w390
            frame "" {
              w451 = ""
            }
            frame Default {
              w457 = " Y%0.3f" ("format string")
              n135 = Scan From String(format string="Y%f", input string=w460) -> (output 1=w456:dbl)  [unwired: 3 in, 3 out]
              n136 = Negate(x=w456) -> (-x=w455:dbl)
              n137 = Add(x=w455, y=w458) -> (x+y=w454:dbl)
              n138 = Format Into String(format string=w457, w455) -> (resulting string=w459:string)  [unwired: 2 in, 1 out]
              n139 = Format Into String(format string=w457, w454) -> (resulting string=w453:string)  [unwired: 2 in, 1 out]
            }
          }
          n140 = case shown="Default" w394 {
            selector: w394 -> [_ w448]
            tunnel: w395 -> [_ w446]
            tunnel: [w439 w447] -> w386
            tunnel: [w439 w441] -> w383
            tunnel: [errorcluster {"status"=TRUE, "code"=0, "source"=""} ("error constant") errorcluster {"status"=FALSE, "code"=0, "source"=""} ("error constant")] -> w391
            frame "" {
              w439 = ""
            }
            frame Default {
              w445 = " Z%0.3f" ("format string")
              n141 = Scan From String(format string="Z%f", input string=w448) -> (output 1=w444:dbl)  [unwired: 3 in, 3 out]
              n142 = Negate(x=w444) -> (-x=w443:dbl)
              n143 = Add(x=w443, y=w446) -> (x+y=w442:dbl)
              n144 = Format Into String(format string=w445, w443) -> (resulting string=w447:string)  [unwired: 2 in, 1 out]
              n145 = Format Into String(format string=w445, w442) -> (resulting string=w441:string)  [unwired: 2 in, 1 out]
            }
          }
          n146 = case shown="Default" w399 {
            selector: w399 -> [_ w472]
            tunnel: w402 -> [_ w470]
            tunnel: [w463 w471] -> w388
            tunnel: [w463 w465] -> w385
            tunnel: [errorcluster {"status"=TRUE, "code"=0, "source"=""} ("error constant") errorcluster {"status"=FALSE, "code"=0, "source"=""} ("error constant")] -> w392
            frame "" {
              w463 = ""
            }
            frame Default {
              w469 = " X%0.3f" ("format string")
              n147 = Scan From String(format string="X%f", input string=w472) -> (output 1=w468:dbl)  [unwired: 3 in, 3 out]
              n148 = Negate(x=w468) -> (-x=w467:dbl)
              n149 = Add(x=w467, y=w470) -> (x+y=w466:dbl)
              n150 = Format Into String(format string=w469, w467) -> (resulting string=w471:string)  [unwired: 2 in, 1 out]
              n151 = Format Into String(format string=w469, w466) -> (resulting string=w465:string)  [unwired: 2 in, 1 out]
            }
          }
          n152 = Merge Errors(w392, w390, w391) -> (w389:errorcluster)
          n153 = Concatenate Strings(w388, w387, w386) -> (w382:string)
          n154 = Concatenate Strings(w385, w384, w383) -> (w381:string)
          n155 = case shown="No Error" w389 {
            selector: w389 -> [w413 _]
            tunnel: w411 -> [w436 _]
            tunnel: w410 -> [w435 _]
            tunnel: w409 -> [w434 _]
            tunnel: w408 -> [w433 _]
            tunnel: w406 -> [w432 _]
            tunnel: w382 -> [w415 _]
            tunnel: w381 -> [w414 _]
            tunnel: [w413 errorcluster {"status"=TRUE, "code"=0, "source"="Error! Format of command is wrong."} ("error constant")] -> w380
            frame No Error {
              w416 = "M501" ("Message")
              w417 = "M500" ("Message")
              w430 = "M210" ("format string")
              w428 = "M211" ("format string")
              # "M211"
              # "M210"
              # "M206"
              n156 = Bundle By Name(cluster=w432, "gCode"=w436, "commandID"=w433) -> (w427:T4)
              n157 = Concatenate Strings(w430, w415) -> (w431:string)
              n158 = Bundle By Name(cluster=w432, "gCode"=w431, "commandID"=w430) -> (w426:T4)
              n159 = call-poly "Enqueue Message.vi"("Message Data"=w427, "Message"=w435, "Message Queue"=w434) -> ("dup Message Queue"=w423:refnum<queue>)  [unwired: 7 in, 1 out]
              n160 = Concatenate Strings(w428, w414) -> (w429:string)
              n161 = Bundle By Name(cluster=w432, "gCode"=w429, "commandID"=w428) -> (w425:T4)
              n162 = call-poly "Enqueue Message.vi"("Message Data"=w426, "Message"=w435, "Message Queue"=w423) -> ("dup Message Queue"=w422:refnum<queue>)  [unwired: 7 in, 1 out]
              n163 = Bundle By Name(cluster=w432, "commandID"=w417, "gCode"=w417) -> (w421:T4)
              n164 = call-poly "Enqueue Message.vi"("Message Data"=w425, "Message"=w435, "Message Queue"=w422) -> ("dup Message Queue"=w424:refnum<queue>)  [unwired: 7 in, 1 out]
              n165 = Bundle By Name(cluster=w432, "commandID"=w416, "gCode"=w416, "extraInfo"="noDisplay") -> (w419:T4)
              n166 = call-poly "Enqueue Message.vi"("Message Data"=w421, "Message"=w435, "Message Queue"=w424) -> ("dup Message Queue"=w420:refnum<queue>)  [unwired: 7 in, 1 out]
              n167 = call-poly "Enqueue Message.vi"("Message Data"=w419, "Message"=w435, "Message Queue"=w420) -> ()  [unwired: 7 in, 2 out]
            }
            frame Error {
            }
          }
        }
        frame "M210" {
          # "Set minimum position --- not allowed to set this property since this will always be 0 plus the home offset (M206)"
        }
        frame "M211" {
          # "Set maximum position  --- set the maximum position assuming that the home position (M206) is zero; thus, set the total travel range. The maximum position shown using M501 is actually the maximum position plus the home offset. The home offset will be automatically added in, so you do not need to worry about it."
          n168 = Two Button Dialog(message="Warning! You should set the maximum travel range here and not the maximum position! The minimum position (M210) is equal to negative the home position (M206) and the maximum position (M211) is equal to the travel range minus the home position. Subtracting away the home position is done automatically; thus, you just need to give the travel range. (For example, as of Oct. 1, 2015, I would use \"M211 X285 Y150 Z150\".) \n \nAre you sure that you want to use your current values to change the maximum position?", 1:"No, let me modify them first." ("F button name (\"Cancel\")"), 2:"Yes, change them." ("T button name (\"OK\")")) -> (T button?=w476:bool)
          n169 = case shown="True" w476 {
            tunnel: w480 -> [_ w495]
            tunnel: w485 -> [_ w494]
            tunnel: w484 -> [_ w492]
            tunnel: w483 -> [_ w491]
            tunnel: w482 -> [_ w490]
            tunnel: w481 -> [_ w489]
            frame False {
            }
            frame True {
              n170 = Unbundle By Name(w495) -> ("pBot_homeOffset"=w487:cluster{"X":dbl, "Y":dbl, "Z":dbl})
              n171 = Match Pattern(string=w494, regular expression="Z[-.0-9]+") -> (match substring=w499:string)  [unwired: 1 in, 3 out]
              n172 = Match Pattern(string=w494, regular expression="Y[-.0-9]+") -> (match substring=w500:string)  [unwired: 1 in, 3 out]
              n173 = Match Pattern(string=w494, regular expression="X[-.0-9]+") -> (match substring=w501:string)  [unwired: 1 in, 3 out]
              n174 = Negate(x=w487) -> (-x=w486:cluster{"X":dbl, "Y":dbl, "Z":dbl})
              n175 = call "flipYZdbl.vi"("pointIn"=w486) -> ("pointOut"=w488:cluster{"X":dbl, "Y":dbl, "Z":dbl})  [unwired: 10 in]
              n176 = Unbundle(w488) -> ("X"=w504:dbl, "Y"=w503:dbl, "Z"=w502:dbl)
              n177 = case shown="Default" w500 {
                selector: w500 -> [_ w536]
                tunnel: w503 -> [_ w532]
                tunnel: ["" w533] -> w498
                frame "" {
                }
                frame Default {
                  n178 = Scan From String(format string="Y%f", input string=w536) -> (output 1=w534:dbl)  [unwired: 3 in, 3 out]
                  n179 = Add(x=w534, y=w532) -> (x+y=w531:dbl)
                  n180 = Format Into String(format string=" Y%0.3f", w531) -> (resulting string=w533:string)  [unwired: 2 in, 1 out]
                }
              }
              n181 = case shown="Default" w499 {
                selector: w499 -> [_ w528]
                tunnel: w502 -> [_ w524]
                tunnel: ["" w525] -> w496
                frame "" {
                }
                frame Default {
                  n182 = Scan From String(format string="Z%f", input string=w528) -> (output 1=w526:dbl)  [unwired: 3 in, 3 out]
                  n183 = Add(x=w526, y=w524) -> (x+y=w523:dbl)
                  n184 = Format Into String(format string=" Z%0.3f", w523) -> (resulting string=w525:string)  [unwired: 2 in, 1 out]
                }
              }
              n185 = case shown="Default" w501 {
                selector: w501 -> [_ w544]
                tunnel: w504 -> [_ w540]
                tunnel: ["" w541] -> w497
                frame "" {
                }
                frame Default {
                  n186 = Scan From String(format string="X%f", input string=w544) -> (output 1=w543:dbl)  [unwired: 3 in, 3 out]
                  n187 = Add(x=w543, y=w540) -> (x+y=w539:dbl)
                  n188 = Format Into String(format string=" X%0.3f", w539) -> (resulting string=w541:string)  [unwired: 2 in, 1 out]
                }
              }
              n189 = Concatenate Strings(w497, w498, w496) -> (w493:string)
              n190 = case shown="Default" w493 {
                selector: w493 -> [_ w519]
                tunnel: w492 -> [_ w520]
                tunnel: w491 -> [_ w512]
                tunnel: w490 -> [_ w513]
                tunnel: w489 -> [_ w521]
                frame "" {
                }
                frame Default {
                  w509 = "M501" ("Message")
                  w510 = "M500" ("Message")
                  n191 = Concatenate Strings(w520, w519) -> (w518:string)
                  n192 = Bundle By Name(cluster=w512, "gCode"=w518, "commandID"=w520) -> (w517:T4)
                  n193 = Bundle By Name(cluster=w512, "gCode"=w510, "commandID"=w510) -> (w515:T4)
                  n194 = Bundle By Name(cluster=w512, "gCode"=w509, "commandID"=w509, "extraInfo"="noDisplay") -> (w511:T4)
                  n195 = call-poly "Enqueue Message.vi"("Message Data"=w517, "Message"=w513, "Message Queue"=w521) -> ("dup Message Queue"=w516:refnum<queue>)  [unwired: 7 in, 1 out]
                  n196 = call-poly "Enqueue Message.vi"("Message Data"=w515, "Message"=w513, "Message Queue"=w516) -> ("dup Message Queue"=w514:refnum<queue>)  [unwired: 7 in, 1 out]
                  n197 = call-poly "Enqueue Message.vi"("Message Data"=w511, "Message"=w513, "Message Queue"=w514) -> ()  [unwired: 7 in, 2 out]
                }
              }
            }
          }
        }
        frame "M212" {
          # "I'm not sure how this one works right now. I might need update yPOI_Home, but for now (Oct 1, 2015) i'll leave this alone."
          # "Set bed probe offset (use this for fine tuning the z-height)"
          n198 = Bundle By Name(cluster=w549, "gCode"=w548, "commandID"=w547) -> (w546:T4)
          n199 = call-poly "Enqueue Message.vi"("Message Data"=w546, "Message"=w550, "Message Queue"=w551) -> ()  [unwired: 7 in, 2 out]
        }
        frame "M502" {
          # "Definately put a pop up window here and confirm the user wants to do this. Should probably also try to save the current values to a text file somewhere."
          # "Resets all tunable parameters to factory reset values."
          n200 = case shown="Default" w558 {
            tunnel: [errorcluster {"status"=TRUE, "code"=0, "source"="Warning! Only one command per line allowed. The first one was used."} ("error constant") errorcluster {"status"=FALSE, "code"=0, "source"=""} ("error constant")] -> w557
            frame Default {
            }
            frame "" {
            }
          }
          n201 = Two Button Dialog(message="This will resent all parameters to the factory default! You will have to reconfigure many things, such as minimum position, maximum position, home offset, max accelerations, etc. Are you sure you want to do this?\n\n(If you do this, then the current settings will first be saved to a file in the applications directory.)", 1:"Cancel" ("F button name (\"Cancel\")"), 2:"Reset" ("T button name (\"OK\")")) -> (T button?=w560:bool)
          n202 = case shown="True" w560 {
            tunnel: w559 -> [_ w566]
            tunnel: w555 -> [_ w569]
            tunnel: w554 -> [_ w571]
            tunnel: w553 -> [_ w573]
            frame False {
            }
            frame True {
              w567 = "M501" ("T button name (\"OK\")")
              # "enqueue first"
              # "enqueue second"
              n203 = Bundle By Name(cluster=w569, "gCode"=w567, "commandID"=w567, "extraInfo"="save" ("T button name (\"OK\")")) -> (w570:T4)
              n204 = call-poly "Enqueue Message.vi"("Message Data"=w570, "Message"=w571, "Message Queue"=w573) -> ("dup Message Queue"=w572:refnum<queue>)  [unwired: 7 in, 1 out]
              n205 = Bundle By Name(cluster=w569, "gCode"=w566, "commandID"=w566) -> (w568:T4)
              n206 = call-poly "Enqueue Message.vi"("Message Data"=w568, "Message"=w571, "Message Queue"=w572) -> ()  [unwired: 7 in, 2 out]
            }
          }
        }
        frame "M501" {
          (unwired) "save" ("extraInfo")
          # "enqueue"
          # "Read parameters from EEPROM"
          n207 = Bundle By Name(cluster=w576, "commandID"=w575, "gCode"=w575) -> (w579:T4)
          n208 = case shown="\"\"" w582 {
            tunnel: [errorcluster {"status"=TRUE, "code"=0, "source"="Warning! Only one command per line allowed. The first one was used."} ("error constant") errorcluster {"status"=FALSE, "code"=0, "source"=""} ("error constant")] -> w581
            frame Default {
            }
            frame "" {
            }
          }
          n209 = call-poly "Enqueue Message.vi"("Message Data"=w579, "Message"=w577, "Message Queue"=w578) -> ()  [unwired: 7 in, 2 out]
        }
        frame "M500" {
          # "enque"
          # "Save parameters to EEPROM"
          n210 = Bundle By Name(cluster=w589, "commandID"=w585, "gCode"=w585) -> (w588:T4)
          n211 = case shown="Default" w592 {
            tunnel: [errorcluster {"status"=TRUE, "code"=0, "source"="Warning! Only one command per line allowed. The first one was used."} ("error constant") errorcluster {"status"=FALSE, "code"=0, "source"=""} ("error constant")] -> w591
            frame Default {
            }
            frame "" {
            }
          }
          n212 = call-poly "Enqueue Message.vi"("Message Data"=w588, "Message"=w587, "Message Queue"=w586) -> ()  [unwired: 7 in, 2 out]
        }
        frame "M600", "M605", "M665", "M668", "M999" {
          # "other commands to ignore"
        }
        frame Default {
          # "IF the command is not in this case structure, then ask the user to make sure they want to send the command to the printerboard"
          n213 = Two Button Dialog(message="The command you entered is not in the list of standard commands. Are you sure that you want to send it to the plasmaBot?", 2:"Send it" ("T button name (\"OK\")")) -> (T button?=w603:bool)  [unwired: 1 in]
          n214 = case shown="True" w603 {
            tunnel: w602 -> [_ w607]
            tunnel: w600 -> [_ w611]
            tunnel: w599 -> [_ w610]
            tunnel: w598 -> [_ w609]
            tunnel: w597 -> [_ w606]
            frame False {
            }
            frame True {
              # "enqueue"
              n215 = Bundle By Name(cluster=w609, "gCode"=w607, "commandID"=w606) -> (w608:T4)
              n216 = call-poly "Enqueue Message.vi"("Message Data"=w608, "Message"=w610, "Message Queue"=w611) -> ()  [unwired: 7 in, 2 out]
            }
          }
        }
      }
    }
    frame True {
      # "Illegal gCode command. I require that a G or M command be the first thing in the string"
    }
  }
  "UI_Data out" <- w7
  "errorOut" <- w6
